vi "Displacement to Global Co-ord.vi"(9 "Angle":dbl, 10 "Displacement y":i16, 11 "Displacement x":i16) -> (2 "Global y":dbl, 3 "Global x":dbl)   [LabVIEW 2012]
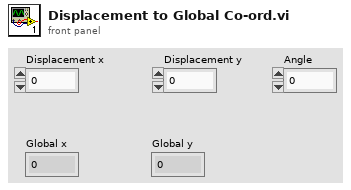
[diagram p1: front panel]
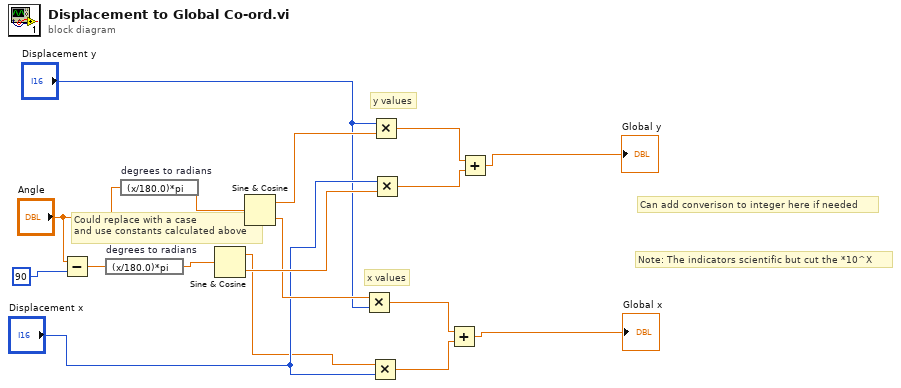
[diagram p0: block diagram]
diagram:
  # "Can add converison to integer here if needed"
  # "Note: The indicators scientific but cut the *10^X"
  # "Could replace with a case\nand use constants calculated above"
  # "x values"
  # "y values"
  n1 = Subtract(x="Angle", y=90) -> (x-y=w7:dbl)
  n2 = expression code="(x/180.0)*pi" "degrees to radians"(w7) -> (w6:dbl)
  n3 = expression code="(x/180.0)*pi" "degrees to radians"("Angle") -> (w17:dbl)
  n4 = Sine & Cosine(0:w6) -> (1:w2:dbl, 2:w5:dbl)
  n5 = Sine & Cosine(0:w17) -> (1:w14:dbl, 2:w4:dbl)
  n6 = Multiply(x=w4, y="Displacement y") -> (x*y=w13:dbl)
  n7 = Multiply(x=w2, y="Displacement x") -> (x*y=w12:dbl)
  n8 = Multiply(x="Displacement y", y=w14) -> (x*y=w16:dbl)
  n9 = Multiply(x="Displacement x", y=w5) -> (x*y=w15:dbl)
  n10 = Add(x=w13, y=w12) -> (x+y=→"Global x":dbl)
  n11 = Add(x=w16, y=w15) -> (x+y=→"Global y":dbl)
